vi "Uniform White Noise.vi"(7 "initialize?":bool=TRUE, 9 "seed":i32=-1, 10 "amplitude":dbl=1.0 format="%0.2f", 11 "samples":i32=128) -> (0 "error":i32, 3 "uniform white noise":dbl[](array[numeric]))   [LabVIEW 2020, in "NI_AALBase.lvlib"]
doc: "Generates a uniformly distributed, pseudorandom pattern whose values are in the range [-a:a], where a is the absolute value of <B>amplitude</B>."
uses:
  NI_AALBase.lvlib
  <resource>/lvanlys.dll
panel:
  # "Uniform White Noise"
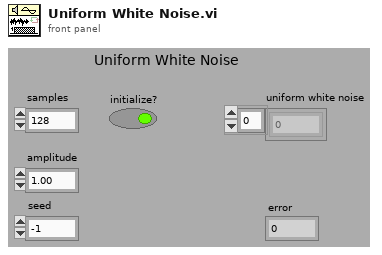
[diagram p1: front panel]
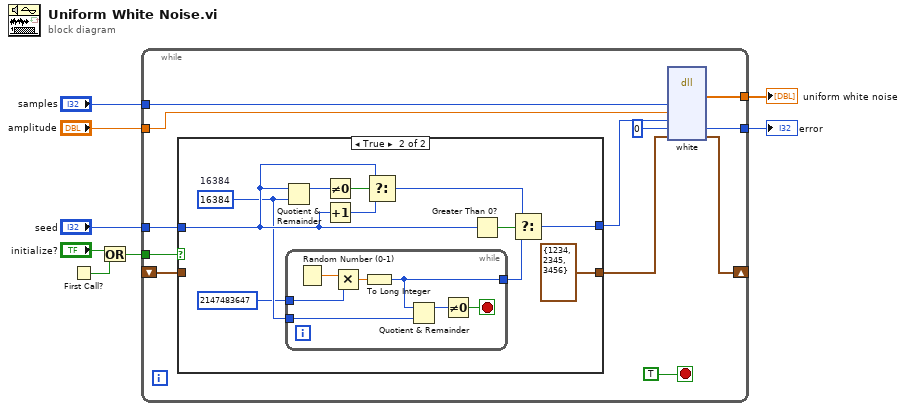
[diagram p0: block diagram]
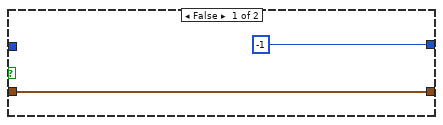
[diagram p2: hidden frame]
diagram:
  n1 = First Call?() -> (First Call?: T/F=w3:bool)
  n2 = Or(x="initialize?", y=w3) -> (x .or. y?=w4:bool)
  n3 = while {
    tunnel: [w20] -> w8
    tunnel: "seed" -> [w14]
    tunnel: "amplitude" -> [w19]
    tunnel: "samples" -> [w18]
    shift-right: [w16] -> _
    shift-left: _ -> [w12]
    tunnel: w4 -> [w13]
    tunnel: [w9] -> w1
    stop <- TRUE stop-if-true
    n4 = case shown="True" w13 {
      tunnel: w12 -> [w22 _]
      tunnel: [w22 cluster{"xSeed":i32, "ySeed":i32, "zSeed":i32} {"xSeed"=1234, "ySeed"=2345, "zSeed"=3456} ("RNGState")] -> w11
      tunnel: [-1 ("seed") w32] -> w10
      tunnel: w14 -> [_ w28]
      frame False {
      }
      frame True {
        w24 = 16384  # 16384
        n5 = Quotient & Remainder(x=w28, y=w24) -> (x-y*floor(x/y)=w30:i32)  [unwired: 1 out]
        n6 = while {
          tunnel: [w38] -> w25
          tunnel: w24 -> [w37]
          tunnel: 2147483647 ("x") -> [w34]
          stop <- w35 stop-if-true
          n7 = Random Number (0-1)() -> (number: 0 to 1=w39:dbl)
          n8 = Multiply(x=w39, y=w34) -> (x*y=w40:dbl)
          n9 = To Long Integer(number=w40) -> (32bit integer=w38:i32)
          n10 = Quotient & Remainder(x=w38, y=w37) -> (x-y*floor(x/y)=w36:i32)  [unwired: 1 out]
          n11 = Not Equal To 0?(x=w36) -> (x != 0?=w35:bool)
        }
        n12 = Not Equal To 0?(x=w30) -> (x != 0?=w29:bool)
        n13 = Increment(x=w28) -> (x+1=w27:i32)
        n14 = Select(t=w28, s=w29, f=w27) -> (s? t:f=w26:i32)
        n15 = Greater Than 0?(x=w28) -> (x > 0?=w33:bool)
        n16 = Select(t=w26, s=w33, f=w25) -> (s? t:f=w32:i32)
      }
    }
    n17 = dll-call lib="C:/Program Files/National Instruments/LabVIEW 2020/resource/lvanlys.*" fn="white"("size"=w18, "ampl"=w19, "theSeed"=w10, "dsperr"=0, "rng_state"=w11) -> ("xH"=w9:dbl[], "dsperr"=w20:i32, "rng_state"=w16:cluster{"xSeed":i32, "ySeed":i32, "zSeed":i32})  [unwired: 6 in, 4 out]
  }
  "error" <- w8
  "uniform white noise" <- w1
